vi "Scan and create Render Stream.vi"(8 "error in":errorcluster, 9 "All Files in Dir":path[](array[path]), 10 "pattern to Include no *":string[](array[string]), 11 "Include vi.lib":bool) -> (0 "error out":errorcluster, 1 "Rendered Stream":string, 2 "Reason":T1(ring), 3 "Is Acyclic ?":bool)   [LabVIEW 2020, in "SimpleDependencyInspector.lvlib"]
uses:
  SimpleDependencyInspector.lvlib
  <vilib>/GraphBuilder/Graph/Graph.lvclass
  <vilib>/GraphBuilder/Node/Node.lvclass
  <vilib>/GraphBuilder/Edge/Edge.lvclass
  <vilib>/GraphBuilder/Renderer/Graphviz/Graphviz.lvclass
  C:/Program Files (x86)/National Instruments/LabVIEW 2020/vi.lib/GraphBuilder/Renderer/Renderer.lvclass
  <vilib>/ProgressBar/Progress Bar Dialog.lvclass
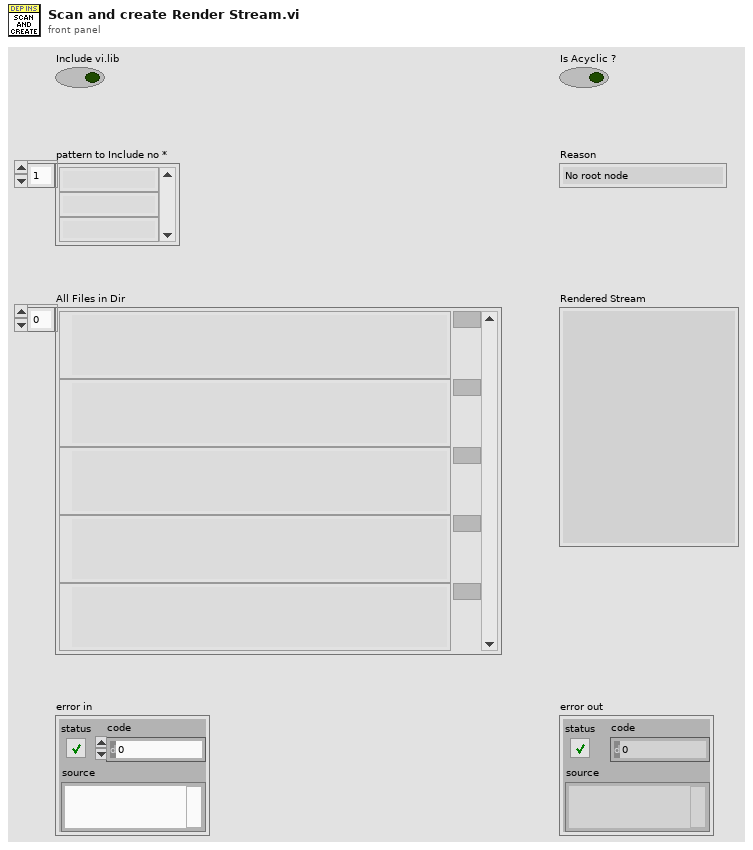
[diagram p1: front panel]
types:
  T1 = enum16{"No root node", "Cycle in graph", "Acyclic", "Error"}
  T2 = typedef "NI_FileType.lvlib/LVFileType.ctl" = enum32{"Invalid file", "Unknown type", "Instrument", "Control", "Polymorphic VI", "Project", "Library", "LVClass", "XControl", "XNode", "Shared library", ".NET assembly", "ActiveX interface", "CIN", "Run-time menu", "Palette menu", "Help file", "LLB", "XNode Edit Dependency", "Class Private Data Control", "Statechart", "MathScript .m file", "Ladder Diagram", "LVLibp", "XNode Build Dependency"}
  T3 = cluster{"path":path, "delimited name":string, "type":T2, "iState":u32, "iStyle":u16, "wStyle":u16, "buttons":u16, "viflags":u32, "viflags2":u32, "links":u32[]}[]
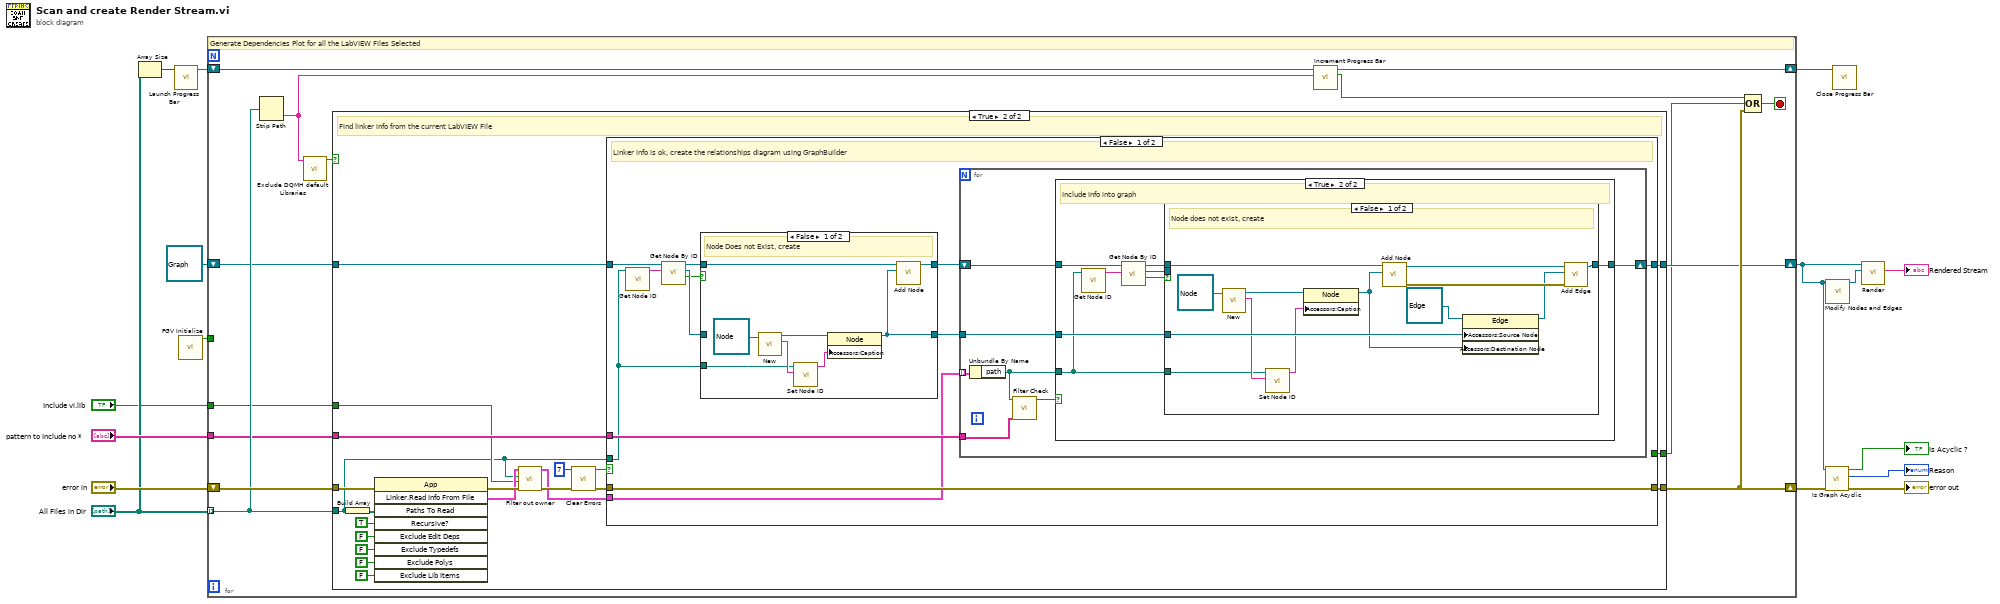
[diagram p0: block diagram]
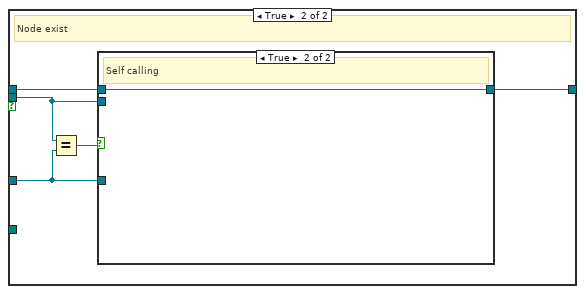
[diagram p4: hidden frame]
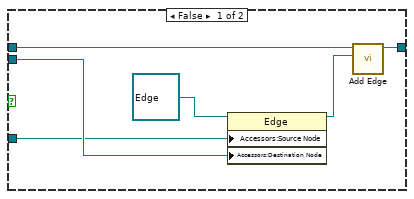
[diagram p5: hidden frame]
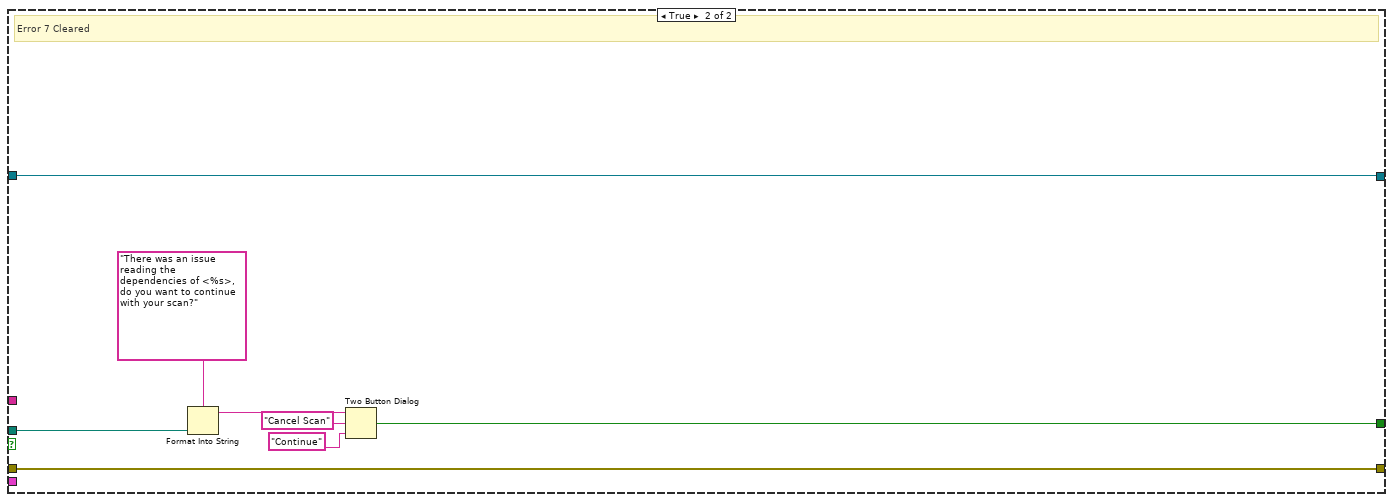
[diagram p7: hidden frame]
diagram:
  n1 = Array Size(array="All Files in Dir") -> (size(s)=w3:i32)
  n2 = call <vilib>:"Launch Progress Bar.vi"("Total Count"=w3) -> ("Progress Bar Dialog"=w2:refnum<class "Progress Bar Dialog.lvclass">)  [unwired: 9 in, 1 out]
  n3 = call "FGV Initialize.vi"() -> ("found?"=w8:bool)  [unwired: 11 in]
  n4 = for {
    shift-right: [w29] -> w15
    shift-left: "error in" -> [w30]
    shift-right: [w27] -> w4
    shift-left: w2 -> [w28]
    tunnel: "All Files in Dir" -> [w26] mode=indexing
    tunnel: "Include vi.lib" -> [w23]
    shift-right: [w21] -> w13
    shift-left: refnum<class "Graph.lvclass"> refnum ("GraphBuilder.lvlib:Graph.lvclass") -> [w20]
    tunnel: w8 -> [_]
    tunnel: "pattern to Include no *" -> [w19]
    stop <- w18 stop-if-true
    # "Generate Dependencies Plot for all the LabVIEW Files Selected"
    n5 = Strip Path(path=w26) -> (name=w22:string)  [unwired: 1 out]
    n6 = call "Exclude DQMH default Libraries.vi"("name"=w22) -> ("Is not a DQMH Default Lib?"=w24:bool)  [unwired: 10 in]
    n7 = case shown="True" w24 {
      tunnel: w30 -> [w32 w53]
      tunnel: [w32 w51] -> w29
      tunnel: w26 -> [_ w33]
      tunnel: w23 -> [_ w34]
      tunnel: [w31 w42] -> w21
      tunnel: w20 -> [w31 w41]
      tunnel: w19 -> [_ w40]
      tunnel: [_ w37] -> w17
      frame False {
        # "Excluding DQMH Template Libraries, this is just to remove noise from the diagram"
      }
      frame True {
        # "Find linker info from the current LabVIEW File"
        n8 = Build Array(w33) -> (w47:path[])
        n9 = invoke class="App" method="Linker.Read Info From File"(error in=w53, "Paths To Read"=w47, "Recursive?"=TRUE, "Exclude Edit Deps"=FALSE ("Exclude Edit Time Dependencies"), "Exclude Typedefs"=FALSE, "Exclude Polys"=FALSE ("Exclude Poly VIs"), "Exclude Lib Items"=FALSE ("Exclude Unused Library Items")) -> (error out=w50:errorcluster, "Linker.Read Info From File"=w36:T3)  [unwired: 2 in, 7 out]
        n10 = call "Filter out owner.vi"("error in"=w50, "Include VI Lib?"=w34, "Owner"=w33, "Linker.Read Info From File in"=w36) -> ("error out"=w49:errorcluster, "Linker.Read Info From File out"=w35:T3)  [unwired: 6 in]
        n11 = call <vilib>:"Clear Errors.vi"("error in (no error)"=w49, "specific error code to clear (0: all)"=7) -> ("error out"=w52:errorcluster, "specific error cleared?"=w38:bool)  [unwired: 4 in]
        n12 = case shown="False" w38 {
          tunnel: [w64 w123] -> w42
          tunnel: w41 -> [w60 w123]
          tunnel: w40 -> [w56 _]
          tunnel: w35 -> [w55 _]
          tunnel: w33 -> [w54 w122]
          tunnel: w52 -> [w65 w124]
          tunnel: [w65 w124] -> w51
          tunnel: [_ w119] -> w37
          frame False {
            # "Linker info is ok, create the relationships diagram using GraphBuilder"
            n13 = call "Get Node ID.vi"("Node Path"=w54) -> ("Node ID"=w61:string)  [unwired: 10 in]
            n14 = call-dynamic "Get Node By ID.vi"("Node ID"=w61, "Graph in"=w60) -> ("Found ?"=w57:bool, "Node"=w58:refnum<class "Node.lvclass">, "Graph out"=w59:refnum<class "Graph.lvclass">)  [unwired: 6 in, 1 out]
            n15 = case shown="False" w57 {
              tunnel: w59 -> [w112 w115]
              tunnel: [w111 w116] -> w63
              tunnel: [w110 w115] -> w62
              tunnel: w58 -> [_ w116]
              tunnel: w54 -> [w107 _]
              frame False {
                # "Node Does not Exist, create"
                n16 = call-dynamic "New.vi"("Node in"=refnum<class "Node.lvclass"> refnum ("Node")) -> ("Node ID"=w109:string, "Node out"=w114:refnum<class "Node.lvclass">)  [unwired: 8 in, 1 out]
                n17 = call "Set Node ID.vi"("Node ID"=w109, "Node Path"=w107) -> ("File Name Out"=w108:string)  [unwired: 9 in]
                n18 = property class="Node"(reference=w114, "Accessors:Caption"=w108) -> (reference out=w111:refnum<class "Node.lvclass">)  [unwired: 1 in, 1 out]
                n19 = call-dynamic "Add Node.vi"("Node"=w111, "Graph in"=w112) -> ("Graph out"=w110:refnum<class "Graph.lvclass">)  [unwired: 8 in, 1 out]
              }
              frame True {
                # "Node Exist, re use"
              }
            }
            n20 = for {
              tunnel: w55 -> [w72] mode=indexing
              shift-right: [w71] -> w64
              shift-left: w62 -> [w70]
              tunnel: w63 -> [w69]
              tunnel: w56 -> [w67]
              n21 = Unbundle By Name(w72) -> ("path"=w66:path)
              n22 = call "Filter Check.vi"("Pattern without asterisk"=w67, "path"=w66) -> ("Include Info"=w68:bool)  [unwired: 9 in]
              n23 = case shown="True" w68 {
                tunnel: w70 -> [w73 w78]
                tunnel: [w73 w81] -> w71
                tunnel: w69 -> [_ w80]
                tunnel: w66 -> [_ w74]
                frame False {
                  # "Include options disable, whether is relative to LabVIEW Instal or it is not included in the plot as file types"
                }
                frame True {
                  # "Include Info into graph"
                  n24 = call "Get Node ID.vi"("Node Path"=w74) -> ("Node ID"=w75:string)  [unwired: 10 in]
                  n25 = call-dynamic "Get Node By ID.vi"("Node ID"=w75, "Graph in"=w78) -> ("Found ?"=w77:bool, "Node"=w76:refnum<class "Node.lvclass">, "Graph out"=w79:refnum<class "Graph.lvclass">)  [unwired: 6 in, 1 out]
                  n26 = case shown="False" w77 {
                    tunnel: [w90 w95] -> w81
                    tunnel: w80 -> [w87 w97]
                    tunnel: w79 -> [w85 w96]
                    tunnel: w76 -> [_ w98]
                    tunnel: w74 -> [w83 _]
                    frame False {
                      # "Node does not exist, create"
                      n27 = call-dynamic "New.vi"("Node in"=refnum<class "Node.lvclass"> refnum ("Node")) -> ("Node ID"=w84:string, "Node out"=w93:refnum<class "Node.lvclass">)  [unwired: 8 in, 1 out]
                      n28 = call "Set Node ID.vi"("Node ID"=w84, "Node Path"=w83) -> ("File Name Out"=w82:string)  [unwired: 9 in]
                      n29 = property class="Node"(reference=w93, "Accessors:Caption"=w82) -> (reference out=w86:refnum<class "Node.lvclass">)  [unwired: 1 in, 1 out]
                      n30 = call-dynamic "Add Node.vi"("Node"=w86, "Graph in"=w85) -> ("error out"=w94:errorcluster, "Graph out"=w91:refnum<class "Graph.lvclass">)  [unwired: 8 in]
                      n31 = property class="Edge"(reference=refnum<class "Edge.lvclass"> refnum ("Edge"), "Accessors:Source Node"=w87, "Accessors:Destination Node"=w86) -> (reference out=w89:refnum<class "Edge.lvclass">)  [unwired: 1 in, 1 out]
                      n32 = call-dynamic "Add Edge.vi"("error in"=w94, "Edge"=w89, "Graph in"=w91) -> ("Graph out"=w90:refnum<class "Graph.lvclass">)  [unwired: 7 in, 1 out]
                    }
                    frame True {
                      # "Node exist"
                      n33 = Equal?(x=w98, y=w97) -> (x = y?=w99:bool)
                      n34 = case shown="True" w99 {
                        tunnel: w98 -> [w105 _]
                        tunnel: w97 -> [w104 _]
                        tunnel: w96 -> [w101 w106]
                        tunnel: [w100 w106] -> w95
                        frame False {
                          n35 = property class="Edge"(reference=refnum<class "Edge.lvclass"> refnum ("Edge"), "Accessors:Source Node"=w104, "Accessors:Destination Node"=w105) -> (reference out=w102:refnum<class "Edge.lvclass">)  [unwired: 1 in, 1 out]
                          n36 = call-dynamic "Add Edge.vi"("Edge"=w102, "Graph in"=w101) -> ("Graph out"=w100:refnum<class "Graph.lvclass">)  [unwired: 8 in, 1 out]
                        }
                        frame True {
                          # "Self calling"
                        }
                      }
                    }
                  }
                }
              }
            }
          }
          frame True {
            # "Error 7 Cleared"
            n37 = Format Into String(format string="There was an issue reading the dependencies of <%s>, do you want to continue with your scan?", w122) -> (resulting string=w120:string)  [unwired: 2 in, 1 out]
            n38 = Two Button Dialog(message=w120, 1:"Continue" ("F button name (\"Cancel\")"), 2:"Cancel Scan" ("F button name (\"Cancel\")")) -> (T button?=w119:bool)
          }
        }
      }
    }
    n39 = call <vilib>:"Increment Progress Bar.vi"("Step Name (\"\")"=w22, "Progress Bar Dialog in"=w28) -> ("Cancelled?"=w25:bool, "Progress Bar Dialog out"=w27:refnum<class "Progress Bar Dialog.lvclass">)  [unwired: 7 in, 1 out]
    n40 = Compound Arithmetic op=OR(w25, w17, w29) -> (w18:bool)
  }
  n41 = call-dynamic "Is Graph Acyclic.vi"("error in"=w15, "Graph in"=w13) -> ("error out"=→"error out":errorcluster, "Reason"=→"Reason":T1, "Is Acyclic ?"=→"Is Acyclic ?":bool)  [unwired: 7 in]
  n42 = call "Modify Nodes and Edges.vi"("Graph in"=w13) -> ("Graphviz out"=w7:refnum<class "Graphviz.lvclass">)  [unwired: 10 in]
  n43 = call <vilib>:"Close Progress Bar.vi"("Progress Bar Dialog"=w4) -> ()  [unwired: 10 in, 1 out]
  n44 = call-dynamic "Render.vi"("Renderer"=w7, "Graph in"=w13) -> ("Rendered Stream"=→"Rendered Stream":string)  [unwired: 7 in, 2 out]
